vi "Write ColorString.vi"(8 "error in (no error)":errorcluster, 10 "ColorString":string, 11 "Paint in":refnum<class "Paint.lvclass">) -> (0 "error out":errorcluster, 3 "Paint out":refnum<class "Paint.lvclass">)   [LabVIEW 2014, in "Paint.lvclass"]
uses:
  Paint.lvclass
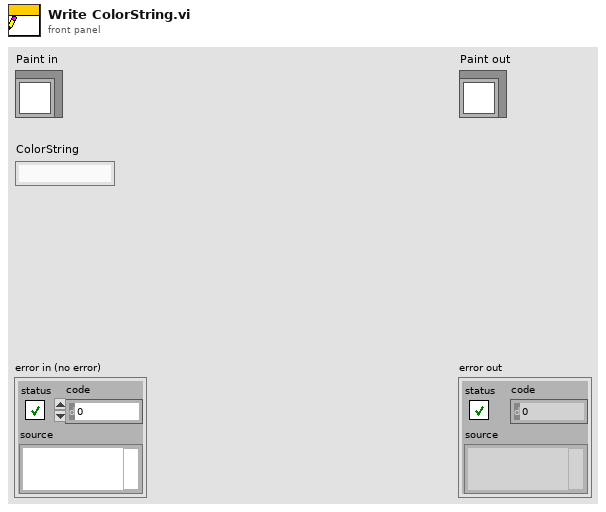
[diagram p1: front panel]
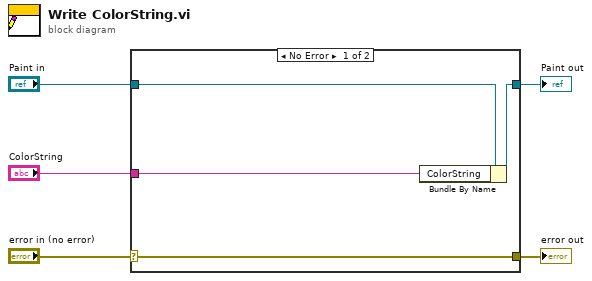
[diagram p0: block diagram]
diagram:
  n1 = case shown="No Error" "error in (no error)" {
    selector: "error in (no error)" -> [w9 w10]
    tunnel: [w9 w10] -> w4
    tunnel: [w7 w11] -> w2
    tunnel: "Paint in" -> [w8 w11]
    tunnel: "ColorString" -> [w6 _]
    frame No Error {
      n2 = Bundle By Name(cluster=w8, "ColorString"=w6) -> (w7:refnum<class "Paint.lvclass">)
    }
    frame Error {
    }
  }
  "error out" <- w4
  "Paint out" <- w2
